vi "S2C_PCIe7841_Proc_ReadSettings.vi"(8 "Error In":errorcluster) -> (0 "Error Out":errorcluster, 3 "ResourceName":string)   [LabVIEW 2015]
doc: "Reads the data contained within the Fornax Commands file and loads the data into the Fornax global variables."
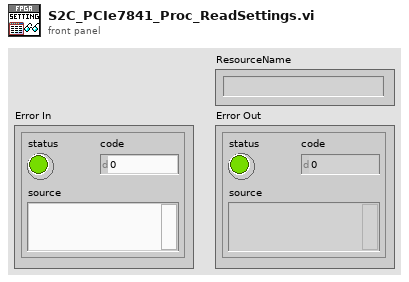
[diagram p1: front panel]
types:
  T1 = enum32{"Bad", "Idle", "Run top level", "Running"}
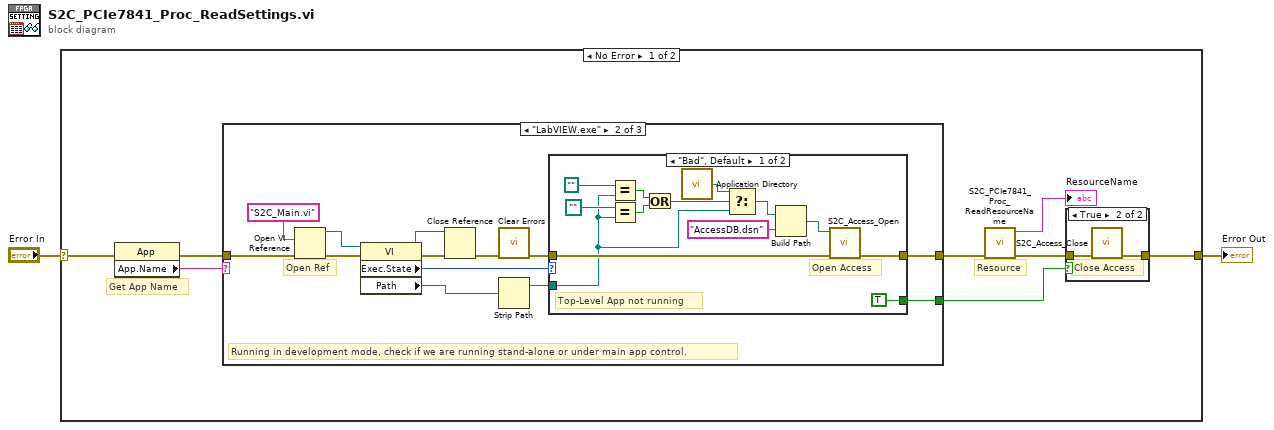
[diagram p0: block diagram]
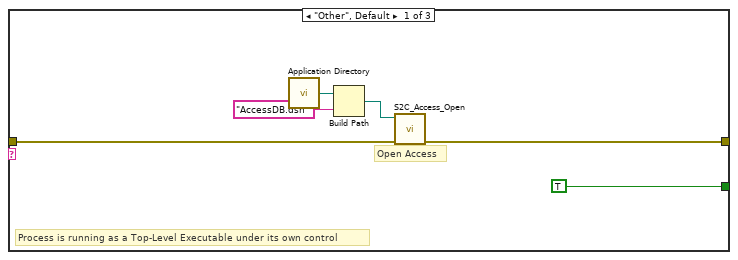
[diagram p2: hidden frame]
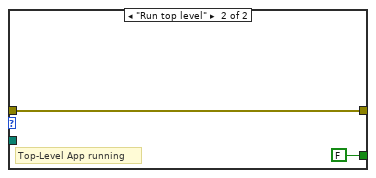
[diagram p3: hidden frame]
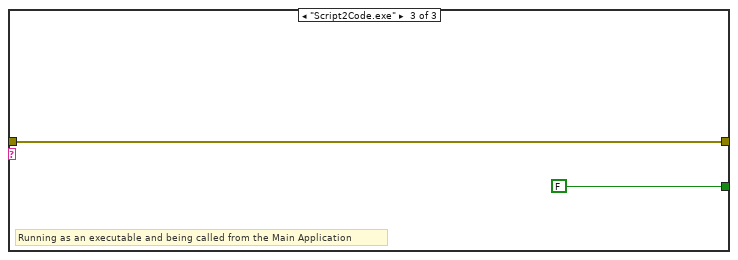
[diagram p4: hidden frame]
diagram:
  n1 = case shown="No Error" "Error In" {
    selector: "Error In" -> [w7 w50]
    tunnel: [w10 w50] -> w1
    frame No Error {
      # "Resource"
      # "Get App Name"
      n2 = property class="App"(error in=w7) -> (error out=w8:errorcluster, "App.Name"=w9:string)  [unwired: 1 in, 1 out]
      n3 = case shown="\"LabVIEW.exe\"" w9 {
        tunnel: w8 -> [w14 w27 w45]
        tunnel: [w12 w24 w45] -> w4
        tunnel: [TRUE ("Exit?") w23 FALSE ("Exit?")] -> w6
        frame "Other", Default {
          # "Open Access"
          # "Process is running as a Top-Level Executable under its own control"
          n4 = call <vilib>:"Application Directory.vi"() -> ("Application Directory"=w15:path)
          n5 = Build Path(base path=w15, name or relative path="AccessDB.dsn") -> (appended path=w13:path)
          n6 = call "S2C_Access_Open.vi"("Error In"=w14, "DSN_Path"=w13) -> ("Error Out"=w12:errorcluster)  [unwired: 8 in, 1 out]
        }
        frame "LabVIEW.exe" {
          # "Running in development mode, check if we are running stand-alone or under main app control."
          # "Open Ref"
          n7 = Open VI Reference(vi path="S2C_Main.vi" ("element"), error in (no error)=w27) -> (vi reference=w28:refnum<vi>, error out=w29:errorcluster)  [unwired: 4 in]
          n8 = property class="VI"(reference=w28, error in=w29) -> (reference out=w21:refnum<vi>, error out=w22:errorcluster, "Exec.State"=w25:T1, "Path"=w18:path)
          n9 = Close Reference(reference=w21, error in (no error)=w22) -> (error out=w20:errorcluster)
          n10 = call <vilib>:"Clear Errors.vi"("error in (no error)"=w20) -> ("error out"=w19:errorcluster)  [unwired: 5 in, 1 out]
          n11 = Strip Path(path=w18) -> (stripped path=w17:path)  [unwired: 1 out]
          n12 = case shown="\"Bad\", Default" w25 {
            tunnel: [w38 w44] -> w24
            tunnel: [TRUE FALSE] -> w23
            tunnel: w19 -> [w39 w44]
            tunnel: w17 -> [w33 _]
            frame "Bad", Default {
              # "Open Access"
              # "Top-Level App not running"
              n13 = Equal?(x=path "", y=w33) -> (x = y?=w32:bool)
              n14 = Equal?(x=path "", y=w33) -> (x = y?=w31:bool)
              n15 = Or(x=w32, y=w31) -> (x .or. y?=w30:bool)
              n16 = call <vilib>:"Application Directory.vi"() -> ("Application Directory"=w36:path)
              n17 = Select(t=w36, s=w30, f=w33) -> (s? t:f=w35:path)
              n18 = Build Path(base path=w35, name or relative path="AccessDB.dsn") -> (appended path=w40:path)
              n19 = call "S2C_Access_Open.vi"("Error In"=w39, "DSN_Path"=w40) -> ("Error Out"=w38:errorcluster)  [unwired: 8 in, 1 out]
            }
            frame "Run top level" {
              # "Top-Level App running"
            }
          }
        }
        frame "Script2Code.exe" {
          # "Running as an executable and being called from the Main Application"
        }
      }
      n20 = call "S2C_PCIe7841_Proc_ReadResourceName.vi"("Error In"=w4) -> ("Error Out"=w5:errorcluster, "ResourceName"=→"ResourceName":string)  [unwired: 9 in]
      n21 = case shown="True" w6 {
        tunnel: w5 -> [w47 w49]
        tunnel: [w47 w48] -> w10
        frame False {
        }
        frame True {
          # "Close Access"
          n22 = call "S2C_Access_Close.vi"("Error In"=w49) -> ("Error Out"=w48:errorcluster)  [unwired: 10 in]
        }
      }
    }
    frame Error {
    }
  }
  "Error Out" <- w1
